vi "Amplitud.vi"(8 "error in (no error)":errorcluster, 10 "Amplitud":dbl, 11 "F Generator in":refnum<class "F Generator.lvclass">) -> (0 "error out":errorcluster, 3 "F Generator out":refnum<class "F Generator.lvclass">)   [LabVIEW 2020, in "F Generator.lvlib" / "F Generator.lvclass"]
uses:
  F Generator.lvclass
  F Generator.lvclass/F Generator.ctl
  Measurement GEN Messages/Amplitud meas Msg/Amplitud meas Msg.lvclass/Amplitud meas Msg.ctl
  <vilib>/ActorFramework/Message Enqueuer/Message Enqueuer.lvclass/Message Enqueuer.ctl
  <vilib>/ActorFramework/Message Enqueuer/Enqueue.vi
  Measurement GEN Messages/Amplitud meas Msg/Amplitud meas Msg.lvclass
  C:/Program Files/National Instruments/LabVIEW 2020/vi.lib/ActorFramework/Message/Message.lvclass
  <vilib>/ActorFramework/Message Priority Queue/Priority Enqueue.vi
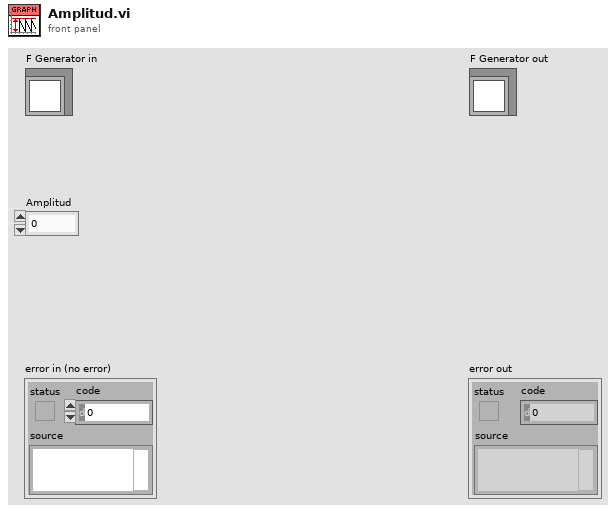
[diagram p1: front panel]
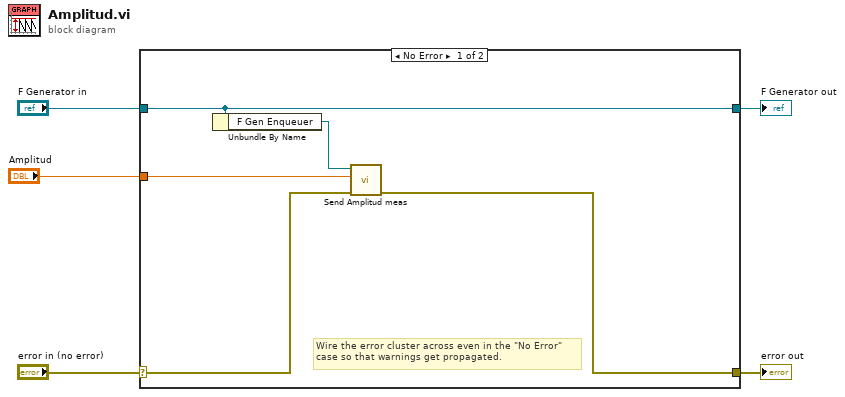
[diagram p0: block diagram]
diagram:
  n1 = case shown="No Error" "error in (no error)" {
    selector: "error in (no error)" -> [w7 w12]
    tunnel: [w6 w12] -> w4
    tunnel: [w10 w11] -> w2
    tunnel: "F Generator in" -> [w10 w11]
    tunnel: "Amplitud" -> [w8 _]
    frame No Error {
      # "Wire the error cluster across even in the \"No Error\"\ncase so that warnings get propagated."
      n2 = Unbundle By Name(w10) -> ("F Gen Enqueuer"=w9:refnum<class "Message Enqueuer.lvclass">)
      n3 = call "Send Amplitud meas.vi"("error in (no error)"=w7, "Amplitud"=w8, "Message Enqueuer"=w9) -> ("error out"=w6:errorcluster)  [unwired: 7 in, 1 out]
    }
    frame Error {
    }
  }
  "error out" <- w4
  "F Generator out" <- w2
